vi "Peaks&Valleys_Finder.vi"(2 "width":i32=3 min=3, 3 "threshold Peaks":dbl format="%0.2f", 4 "waveform in":waveform(dbl)) -> (0 "Amplitudes Peaks":dbl[](array[numeric]), 1 "Locations Peaks":dbl[](array[numeric]))   [LabVIEW 2024]
uses:
  <vilib>/measure/mamon.llb/Waveform Peak Detection for 1 Chan.vi
  <vilib>/measure/NI_MAPro.lvlib
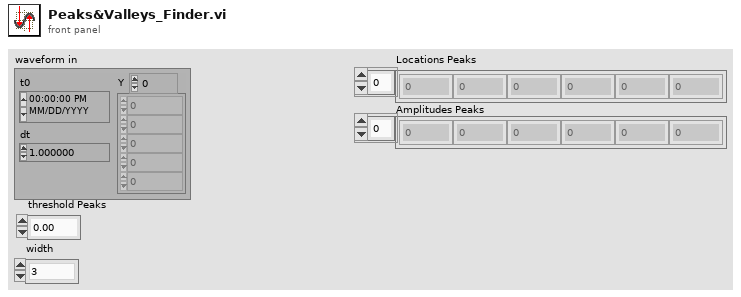
[diagram p1: front panel]
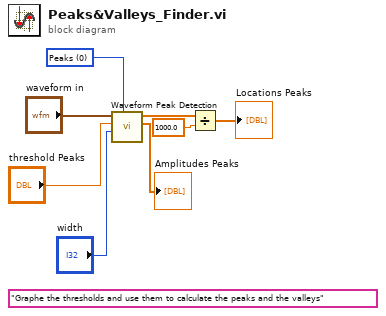
[diagram p0: block diagram]
diagram:
  w5 = u16 0 items=["Peaks", "Valleys"] ("peaks/valleys")
  (unwired) "Graphe the thresholds and use them to calculate the peaks and the valleys"
  n1 = call-poly <vilib>:"Waveform Peak Detection.vi"("peaks/valleys"=w5, "width"="width", "threshold"="threshold Peaks", "Signal In"="waveform in") -> ("Amplitudes"=→"Amplitudes Peaks":dbl[], "Locations"=w2:dbl[])  [unwired: 3 in, 3 out]
  n2 = Divide(x=w2, y=1000.0) -> (x/y=→"Locations Peaks":dbl[])
